vi "Priority.vi"(8 "error in (no error)":errorcluster, 11 "Session Response Handler in":refnum<class "Session Response Handler.lvclass">) -> (0 "error out":errorcluster, 2 "Priority":u16, 3 "Session Response Handler out":refnum<class "Session Response Handler.lvclass">)   [LabVIEW 2020, in "HTTP Server.lvlib" / "Session Response Handler.lvclass"]
uses:
  Session Response Handler.lvclass
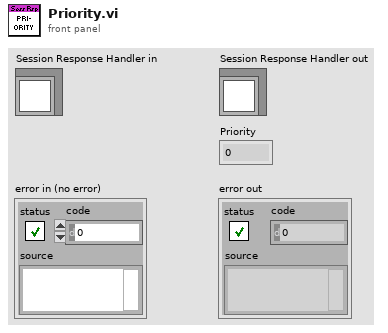
[diagram p1: front panel]
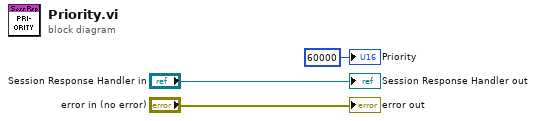
[diagram p0: block diagram]
diagram:
  "error out" <- "error in (no error)"
  "Session Response Handler out" <- "Session Response Handler in"
  "Priority" <- u16 60000 ("Priority")
